vi "InitializeShotTimeArray.vi"(1 "InvaderArray":bool[][](array[boolean])) -> (0 "InvaderColoumnTimeArray":u32[](array[numeric]))   [LabVIEW 2022 SP3]
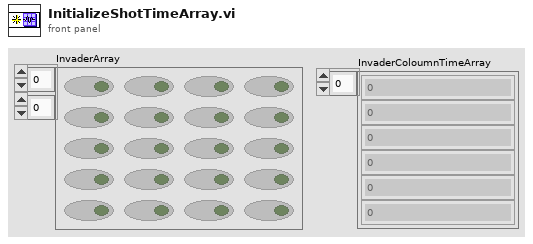
[diagram p1: front panel]
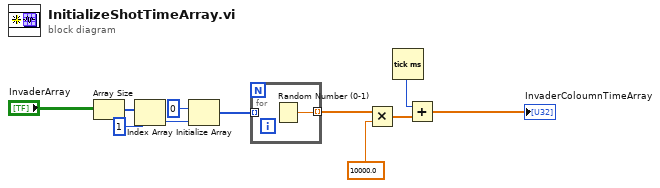
[diagram p0: block diagram]
diagram:
  n1 = Array Size(array="InvaderArray") -> (size(s)=w8:i32[])
  n2 = Index Array(array=w8, index=1) -> (element=w11:i32)
  n3 = Initialize Array(u32 0 ("element"), w11) -> (w6:u32[])
  n4 = for {
    tunnel: w6 -> [_] mode=indexing
    tunnel: [w12] -> w4 mode=indexing
    n5 = Random Number (0-1)() -> (number: 0 to 1=w12:dbl)
  }
  n6 = Multiply(x=w4, y=10000.0) -> (x*y=w5:dbl[])
  n7 = Tick Count (ms)() -> (millisecond timer value=w2:u32)
  n8 = Add(x=w2, y=w5) -> (x+y=→"InvaderColoumnTimeArray":dbl[])
